vi "ReadBAESdataFromFileMCVersion.vi"(0 "file path":path) -> (1 "Extinction ExtinctionUncertainity Size parameter and Number ofS sizes":T1, 2 "FullExtinctionData":dbl[][](array[numeric]), 3 "NumberOfMeasurementsperSize":i32)   [LabVIEW 2013]
uses:
  ReadBaesDataTypeDefinition.ctl
  <vilib>/Platform/storage/lvStorage.llb/_openStorageWithRootAutoDetect.vi
  <vilib>/Platform/storage/lvStorage.llb/xStorage/xStorageSupp/ErrorOut.vi
  <vilib>/Platform/storage/lvStorage.llb/_queryPropPoly.vi
  <vilib>/Platform/storage/lvStorage.llb/_queryPropString.vi
  <vilib>/Platform/storage/lvStorage.llb/_queryGenericObjects.vi
  <vilib>/Platform/storage/lvStorage.llb/_loadAllDouble.vi
  <vilib>/Platform/storage/Storage.llb/Get Object Info.vi
  <vilib>/Platform/storage/Storage.llb/__closeStorageFromObject.vi
  <vilib>/imath/engines/lvmath2/RunTimeEngine/ErrorHandling/NIMS_Finalize Error.vi
  <vilib>/imath/engines/lvmath2/RunTimeEngine/Managers/WorkSpace/UID Generator.vi
  <vilib>/imath/engines/lvmath2/RunTimeEngine/Managers/SymbolTable/Clear UID.vi
  <vilib>/imath/engines/lvmath2/RunTimeEngine/NodeEndStatement/NIMS_NodeEndStatement_Output.vi
  <instcachedir>/0/NIMS_NodeEndStatement_Output_53EC0D466D134D7ABD903AC30B43404B.lvgen/NIMS_NodeEndStatement_Output_53EC0D466D134D7ABD903AC30B43404B_010.vi
  <instcachedir>/0/NIMS_NodeEndStatement_Output_53EC0D466D134D7ABD903AC30B43404B.lvgen/NIMS_NodeEndStatement_Output_53EC0D466D134D7ABD903AC30B43404B_002.vi
  <instcachedir>/0/NIMS_NodeEndStatement_Output_53EC0D466D134D7ABD903AC30B43404B.lvgen/NIMS_NodeEndStatement_Output_53EC0D466D134D7ABD903AC30B43404B_005.vi
  <vilib>/imath/engines/lvmath2/RunTimeEngine/IndexRead/NIMS M(S,S).vi
  <instcachedir>/0/NIMS M(S,S)_AC51E74150A542F7991B9634C66F3096.lvgen/NIMS M(S,S)_AC51E74150A542F7991B9634C66F3096_000.vi
  <vilib>/imath/engines/lvmath2/RunTimeEngine/IndexRead/NIMS M(S,R2).vi
  <instcachedir>/0/NIMS M(S,R2)_45730E4D0DB74D118F715F4F99DCE4D7.lvgen/NIMS M(S,R2)_45730E4D0DB74D118F715F4F99DCE4D7_000.vi
  <vilib>/imath/engines/lvmath2/RunTimeEngine/BuiltInFunctions/findnz/NIMS_[1o]_findnz(GRowV).vi
  <instcachedir>/0/NIMS_[1o]_findnz(GRowV)_A907680C39E74AF18CBD76E991AC1137.lvgen/NIMS_[1o]_findnz(GRowV)_A907680C39E74AF18CBD76E991AC1137_000.vi
  <vilib>/imath/engines/lvmath2/RunTimeEngine/BuiltInFunctions/length/NIMS_length(GV).vi
  <instcachedir>/0/NIMS_length(GV)_08A3D13377FD4E4B96F5795FBF3698FA.lvgen/NIMS_length(GV)_08A3D13377FD4E4B96F5795FBF3698FA_002.vi
  <vilib>/imath/engines/lvmath2/RunTimeEngine/RunTimeType/NIMS_RunTimeType_From StrictType (excl LVString).vi
  <instcachedir>/0/NIMS_RunTimeType_From StrictType (excl LVString)_4DEE718D6EB74582AA20236969C084FC.lvgen/NIMS_RunTimeType_From StrictType (excl LVString)_4DEE718D6EB74582AA20236969C084FC_000.vi
  <vilib>/imath/engines/lvmath2/RunTimeEngine/LocalVariableDefStatement/MC_LocalVariableDefStatement_Display.vi
  <vilib>/imath/engines/lvmath2/RunTimeEngine/ErrorHandling/NIMS_Create Error From Enums.vi
  <vilib>/imath/engines/lvmath2/RunTimeEngine/IndexRead/NIMS M(S,$).vi
  <instcachedir>/0/NIMS M(S,$)_F24F360562DE41D8BE234322A2E15C65.lvgen/NIMS M(S,$)_F24F360562DE41D8BE234322A2E15C65_000.vi
  <instcachedir>/0/NIMS_length(GV)_08A3D13377FD4E4B96F5795FBF3698FA.lvgen/NIMS_length(GV)_08A3D13377FD4E4B96F5795FBF3698FA_000.vi
  <vilib>/imath/engines/lvmath2/RunTimeEngine/IndexRead/NIMS M(S,R3).vi
  <instcachedir>/0/NIMS M(S,R3)_3691D2D1C76942D2AB3524405DAA5FED.lvgen/NIMS M(S,R3)_3691D2D1C76942D2AB3524405DAA5FED_000.vi
  <vilib>/imath/engines/lvmath2/RunTimeEngine/IndexRead/NIMS M(R2,S).vi
  <instcachedir>/0/NIMS M(R2,S)_56813DCFDD5A484292D2195AF15D2BF5.lvgen/NIMS M(R2,S)_56813DCFDD5A484292D2195AF15D2BF5_000.vi
  <vilib>/imathl/engines/lvmath/Functions/Error Handling/Create Error.vi
  <vilib>/imath/engines/lvmath2/RunTimeEngine/RangeToken/NIMS_Range_R3 - Integer.vi
  <instcachedir>/0/NIMS_Range_R3 - Integer_61C6A1A9DF45400FA53C335A664ED8E6.lvgen/NIMS_Range_R3 - Integer_61C6A1A9DF45400FA53C335A664ED8E6_000.vi
  <vilib>/imath/engines/lvmath2/RunTimeEngine/CommandStatement/MC_CommandStatement_break.vi
  <vilib>/imath/engines/lvmath2/RunTimeEngine/IndexRead/NIMS M(R2,R2).vi
  <instcachedir>/0/NIMS M(R2,R2)_A604CBC2A3B94D18B31C03B21D5CD7AA.lvgen/NIMS M(R2,R2)_A604CBC2A3B94D18B31C03B21D5CD7AA_000.vi
  <vilib>/imath/engines/lvmath2/RunTimeEngine/BuiltInFunctions/mean/NIMS_RCol=mean(RM,I32).vi
  <vilib>/imath/engines/lvmath2/RunTimeEngine/RowToken/NIMS_RowToken_M_CV.vi
  <instcachedir>/0/NIMS_RowToken_M_CV_4FFFB80A1A2C4A06BEF1E2564C6BAFA4.lvgen/NIMS_RowToken_M_CV_4FFFB80A1A2C4A06BEF1E2564C6BAFA4_000.vi
  <vilib>/imath/engines/lvmath2/RunTimeEngine/BuiltInFunctions/std/NIMS_std(GM,RV).vi
  <instcachedir>/0/NIMS_std(GM,RV)_76610E1FBF9A4039B8A2AB91E88BA79F.lvgen/NIMS_std(GM,RV)_76610E1FBF9A4039B8A2AB91E88BA79F_001.vi
  <vilib>/imath/engines/lvmath2/RunTimeEngine/MatrixToken/NIMS_MatrixToken_M_RV.vi
  <instcachedir>/0/NIMS_MatrixToken_M_RV_B5D6FED72B2644F1B51E8342DCF604DF.lvgen/NIMS_MatrixToken_M_RV_B5D6FED72B2644F1B51E8342DCF604DF_001.vi
  <vilib>/imath/engines/lvmath2/RunTimeEngine/BuiltInFunctions/repeatmx/NIMS_repeatmx(GM, I32, I32).vi
  <instcachedir>/0/NIMS_repeatmx(GM, I32, I32)_71D32CAC8D434697AB9DA7B55FCB46E4.lvgen/NIMS_repeatmx(GM, I32, I32)_71D32CAC8D434697AB9DA7B55FCB46E4_000.vi
  <vilib>/imath/engines/lvmath2/RunTimeEngine/ArithmeticOperatorToken/NIMS_ArithmeticOperator_rightdiv.vi
  <instcachedir>/0/NIMS_ArithmeticOperator_rightdiv_C75411BD8BC84A93B6F1C8DA359A92EC.lvgen/NIMS_ArithmeticOperator_rightdiv_C75411BD8BC84A93B6F1C8DA359A92EC_004.vi
  <vilib>/Platform/storage/lvStorage.llb/xStorage/Open Data Storage/Open Data Storage.xnode
  <vilib>/Platform/storage/lvStorage.llb/xStorage/Read Data/Read Data.xnode
  <vilib>/Platform/storage/lvStorage.llb/xStorage/Close Data Storage/Close Data Storage.xnode
  <vilib>/imath/engines/lvmath2/RunTimeEngine/Managers/SymbolTable/NIMS_WorkSpace.lvlib
panel:
  in  "Extinction ExtinctionUncertainity Size parameter and Number ofS sizes 2":T1
  out "Signal":dbl[][](array[numeric])
  out "GeometricCrossSection":dbl[](array[numeric])
  out "Number Of Sizes":dbl
  out "SizeParameter":dbl[][](array[numeric])
  in  "Slide":i16(slide) scale=0.0..100.0
  out "Extinction Graph":cluster{"Extinction":dbl[], "Sizes":dbl[]}[](graph)
  out "ExtinctionUncertainty":dbl[][](array[numeric])
  out "Extinction":dbl[][](array[numeric])
  out "WaveLengths":dbl[](array[numeric])
  out "error out":errorcluster
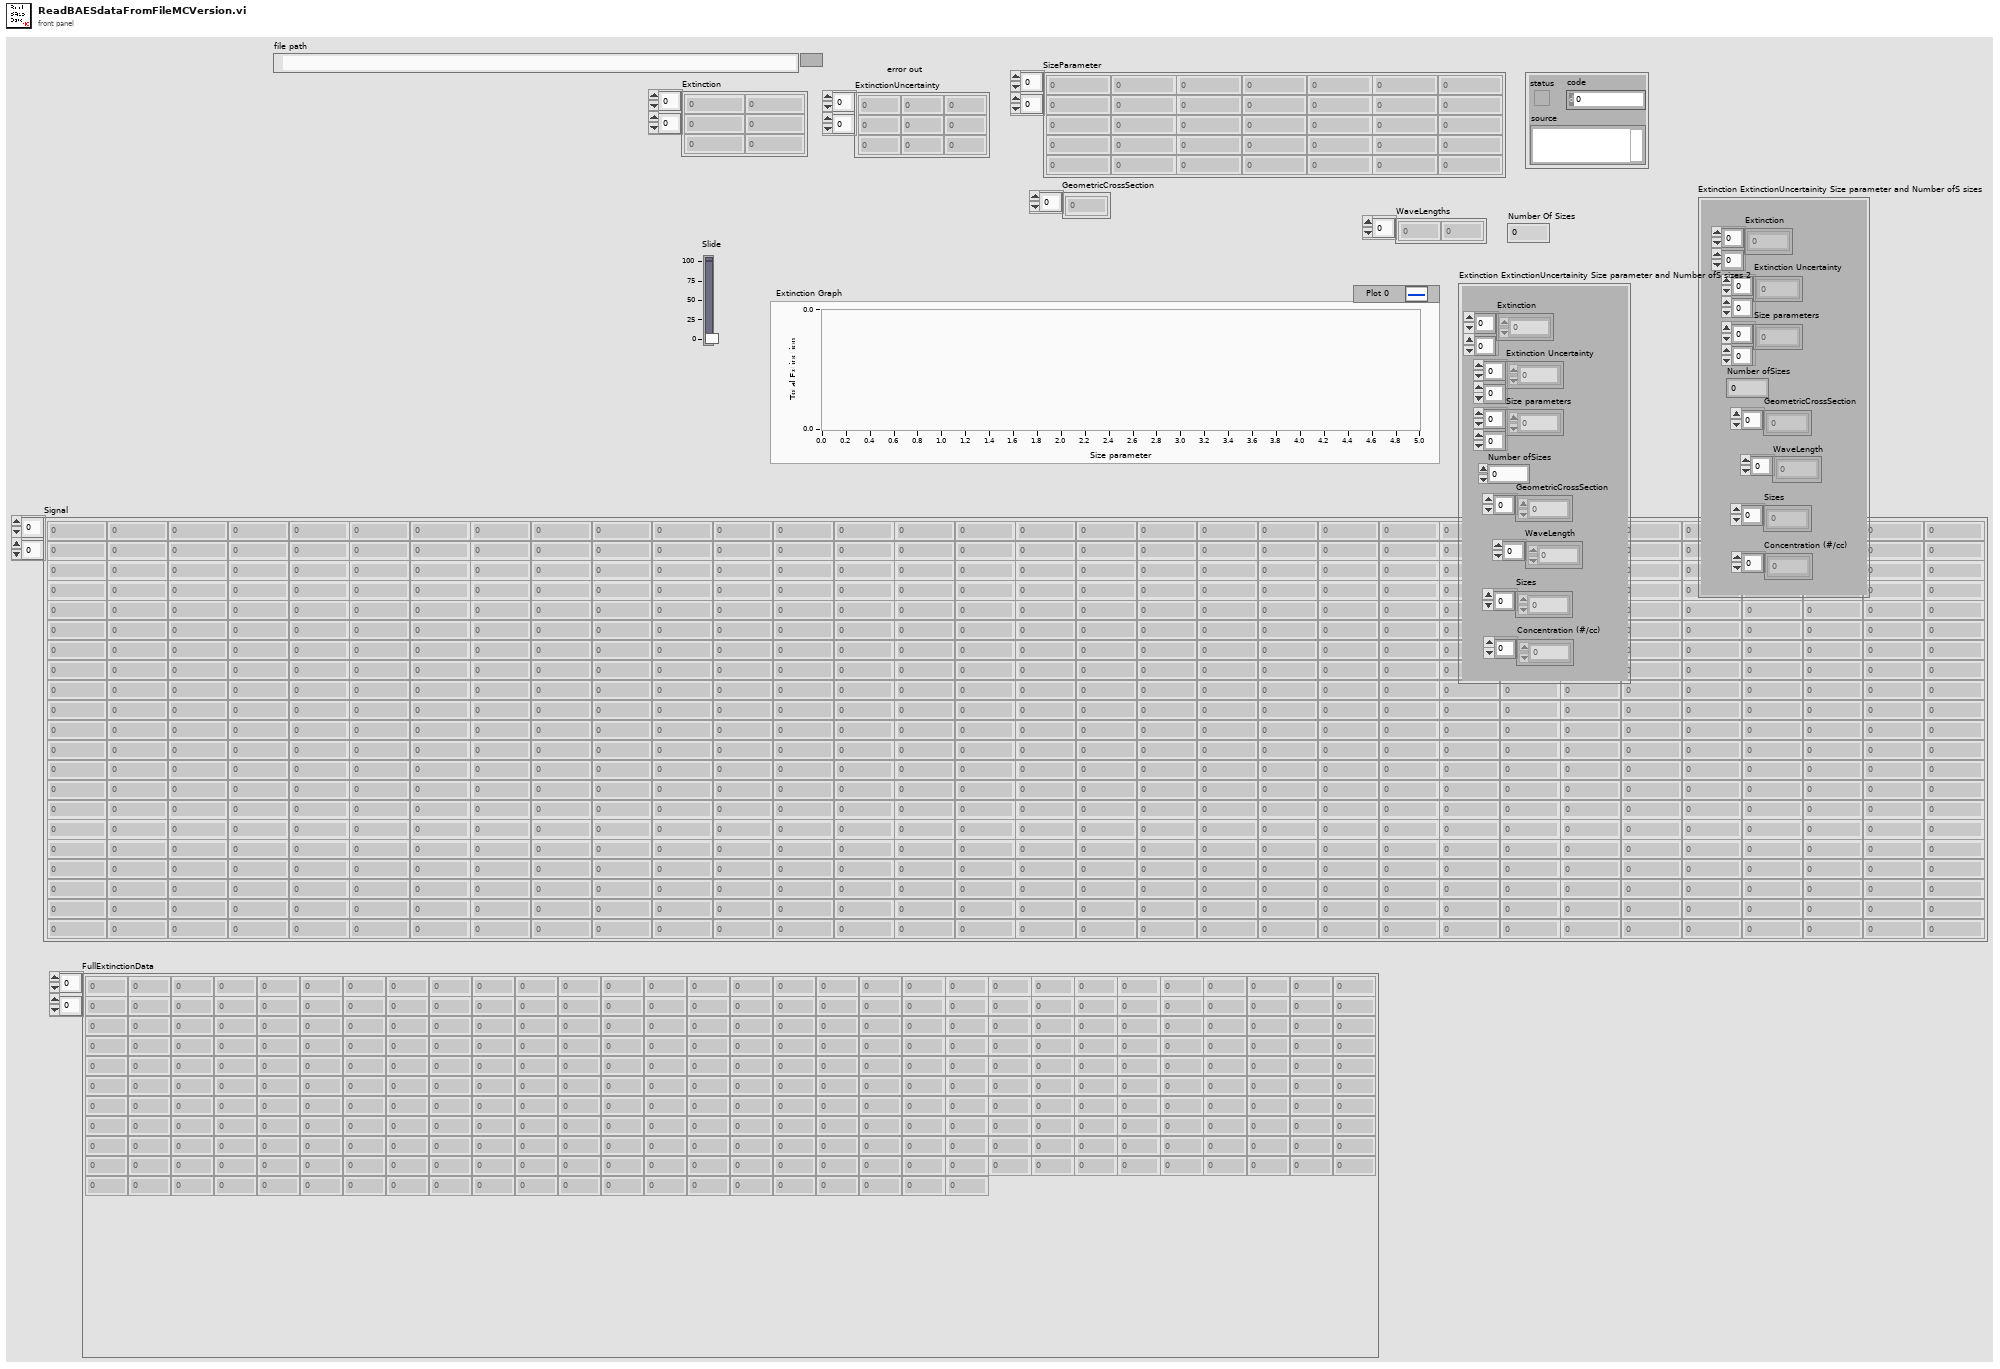
[diagram p1: front panel]
types:
  T1 = typedef "ReadBaesDataTypeDefinition.ctl" = cluster{"Extinction":dbl[][], "Extinction Uncertainty":dbl[][], "Size parameters":dbl[][], "Number ofSizes":dbl, "GeometricCrossSection":dbl[], "WaveLength":dbl[], "Sizes":dbl[], "Concentration (#/cc)":dbl[]}
  T2 = enum16{"open", "open or create", "create or replace", "create", "open (read only)"}
  T3 = cluster{"SizeParameter":dbl[], "Extinction":dbl[]}
  T4 = cluster{"SizeParameter":dbl[], "Extinction":dbl[]}[]
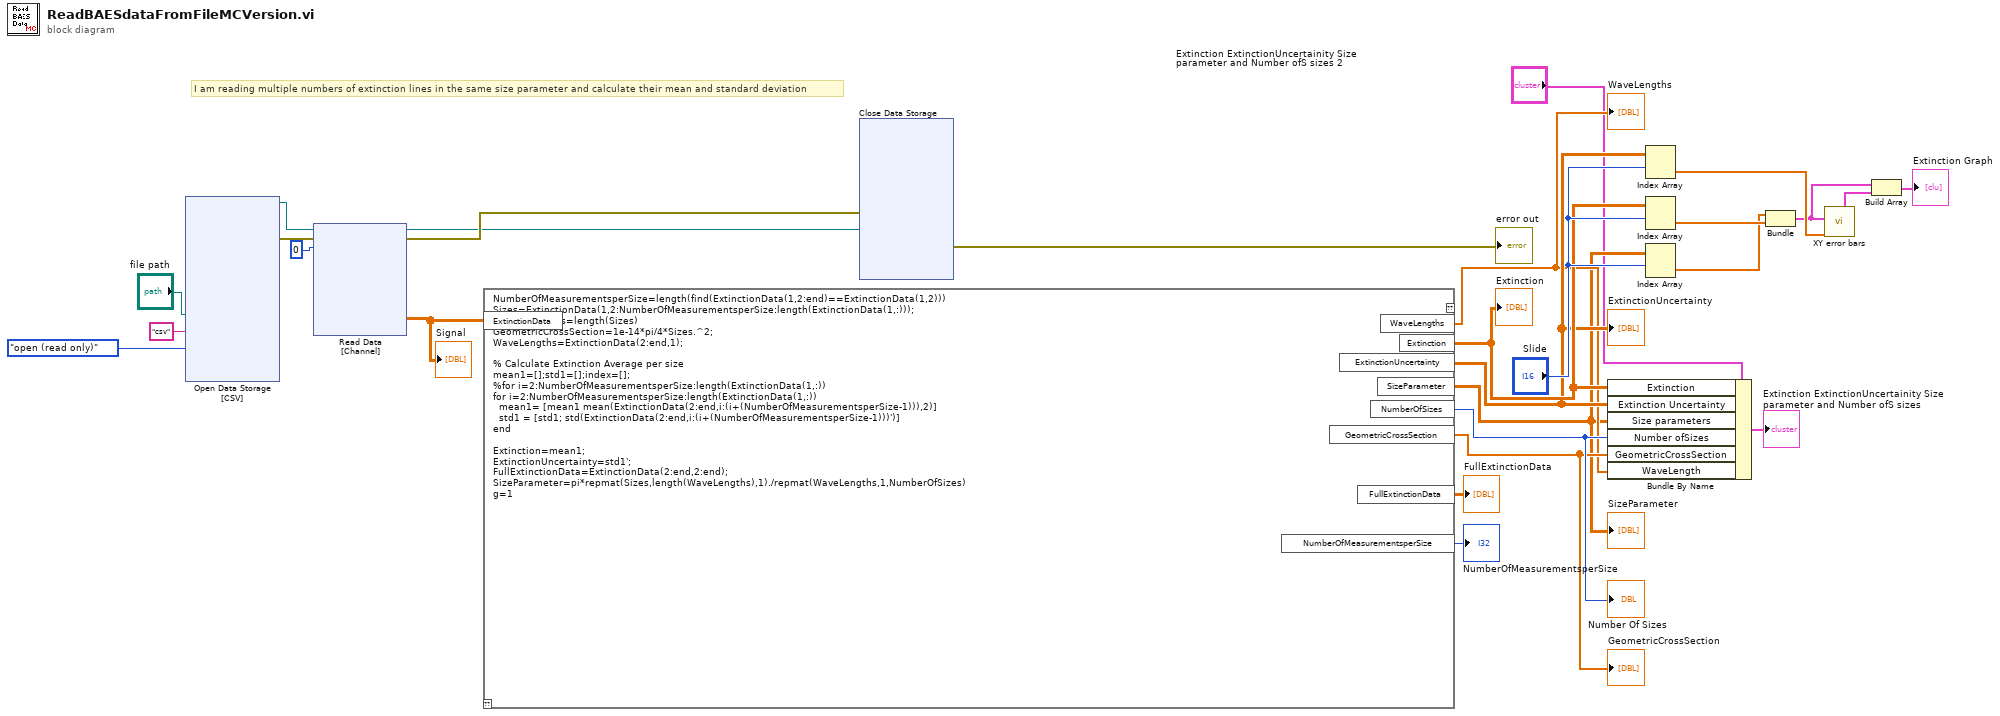
[diagram p0: block diagram]
diagram:
  # "I am reading multiple numbers of extinction lines in the same size parameter and calculate their mean and standard deviation"
  n1 = xnode "Open Data Storage\n[CSV]"("file path"="file path", "DataPlugin name"="csv", "function (open:0)"=T2."open (read only)") -> ("storage refnum (file)"=w27:refnum<k20>, "error out"=w26:errorcluster)  [unwired: 2 in, 1 out]
  n2 = xnode "Read Data\n[Channel]"("storage refnum (file)"=w27, "error in"=w26, "index"=0) -> ("Signal"=w13:dbl[][], "storage refnum (file) out"=w21:refnum<k20>, "error out"=w25:errorcluster)  [unwired: 1 in, 1 out]
  "Signal" <- w13
  n3 = mathscript code="NumberOfMeasurementsperSize=length(find(ExtinctionData(1,2:end)==ExtinctionData(1,2)))\nSizes=ExtinctionData(1,2:NumberOfMeasurementsperSize:length(ExtinctionData(1,:)));\nNumberOfSizes=length(Sizes)\nGeometricCrossSection=1e-14*pi/4*Sizes.^2;\nWaveLengths=ExtinctionData(2:end,1);\n\n% Calculate Extinction Average per size\nmean1=[];std1=[];index=[];\n%for i=2:NumberOfMeasurementsperSize:length(ExtinctionData(1,:))\nfor i=2:NumberOfMeasurementsperSize:length(ExtinctionData(1,:))\n  mean1= [mean1 mean(ExtinctionData(2:end,i:(i+(NumberOfMeasurementsperSize-1))),2)]\n  std1 = [std1; std(ExtinctionData(2:end,i:(i+(NumberOfMeasurementsperSize-1)))')]\nend\n\nExtinction=mean1;\nExtinctionUncertainty=std1';\nFullExtinctionData=ExtinctionData(2:end,2:end);\nSizeParameter=pi*repmat(Sizes,length(WaveLengths),1)./repmat(WaveLengths,1,NumberOfSizes)\ng=1"("ExtinctionData"=w13) -> ("WaveLengths"=w6:dbl[], "Extinction"=w10:dbl[][], "ExtinctionUncertainty"=w9:dbl[][], "SizeParameter"=w5:dbl[][], "NumberOfSizes"=w8:i32, "GeometricCrossSection"=w7:dbl[], "FullExtinctionData"=→"FullExtinctionData":dbl[][], "NumberOfMeasurementsperSize"=→"NumberOfMeasurementsperSize":i32)  [unwired: 1 in, 1 out]
  "WaveLengths" <- w6
  "Extinction" <- w10
  "ExtinctionUncertainty" <- w9
  "SizeParameter" <- w5
  "Number Of Sizes" <- w8
  "GeometricCrossSection" <- w7
  n4 = xnode "Close Data Storage\n"("error in (no error)"=w25, "storage refnum (file)"=w21) -> ("error out"=→"error out":errorcluster)  [unwired: 1 out]
  n5 = Bundle By Name(cluster="Extinction ExtinctionUncertainity Size parameter and Number ofS sizes 2", "Extinction"=w10, "Extinction Uncertainty"=w9, "Size parameters"=w5, "Number ofSizes"=w8, "GeometricCrossSection"=w7, "WaveLength"=w6) -> (→"Extinction ExtinctionUncertainity Size parameter and Number ofS sizes":T1)
  n6 = Index Array(array=w9, index (row)="Slide") -> (element=w20:dbl[])  [unwired: 1 in]
  n7 = Index Array(array=w10, index (row)="Slide") -> (element=w16:dbl[])  [unwired: 1 in]
  n8 = Index Array(array=w5, index (row)="Slide") -> (element=w14:dbl[])  [unwired: 1 in]
  n9 = Bundle("SizeParameter"=w14, "Extinction"=w16) -> (w19:T3)  [unwired: 1 in]
  n10 = call "XY error bars.vi"("XY plot"=w19, "Yerror"=w20) -> ("Y error bars"=w18:cluster{dbl[], dbl[]})  [unwired: 6 in, 2 out]
  n11 = Build Array(w19, w18) -> (→"Extinction Graph":T4)
